vi "Get settings chain.vi"(8 "error in (no error)":errorcluster, 11 "ConfocalStageBase in":refnum<class "ConfocalStage.lvclass">) -> (0 "error out":errorcluster, 1 "class name":string[](array[string]), 2 "settings":variant[](array[variant]), 3 "ConfocalStageBase out":refnum<class "ConfocalStage.lvclass">)   [LabVIEW 2012, in "ConfocalStage.lvclass"]
doc: "Returns an array of variants containing the settings clusters of each class in the inheritance chain (lowest child class first), together with an array of all class names in the inheritance chain.\n\nFor classes without settings cluster, the settings chain contains empty variants."
uses:
  ConfocalStage.lvclass
  <vilib>/Distrio/Murmex/Murmex/Murmex.lvclass
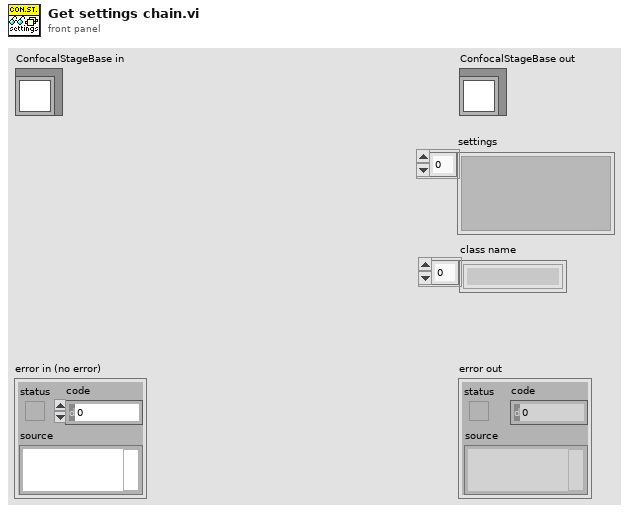
[diagram p1: front panel]
types:
  T1 = typedef "ConfocalStage.lvclass/settings.ctl" = cluster{"X stage speed":dbl, "Y stage speed":dbl, "Z stage speed":dbl}
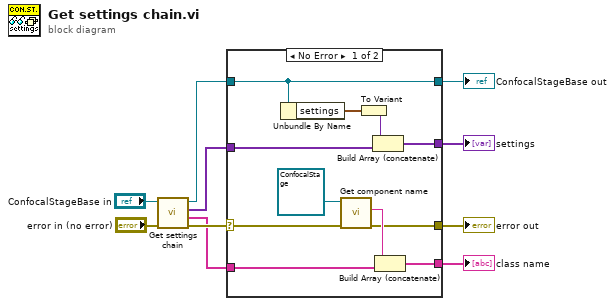
[diagram p0: block diagram]
diagram:
  n1 = call-parent "Get settings chain.vi"("error in (no error)"="error in (no error)", "MurmexBase in"="ConfocalStageBase in") -> ("error out"=w8:errorcluster, "class name"=w3:string[], "settings"=w4:variant[], "MurmexBase out"=w6:refnum<class "ConfocalStage.lvclass">)  [unwired: 6 in]
  n2 = case shown="No Error" w8 {
    selector: w8 -> [w18 w22]
    tunnel: [w17 w22] -> w7
    tunnel: w6 -> [w16 w23]
    tunnel: [w16 w23] -> w5
    tunnel: w4 -> [w15 _]
    tunnel: w3 -> [w14 _]
    tunnel: [w12 _] -> w2
    tunnel: [w11 _] -> w1
    frame No Error {
      n3 = Unbundle By Name(w16) -> ("settings"=w20:T1)
      n4 = call <vilib>:"Get component name.vi"("error in (no error)"=w18, "Murmex in"=refnum<class "ConfocalStage.lvclass"> refnum ("ConfocalStageBase in")) -> ("error out"=w17:errorcluster, "component name"=w19:string)  [unwired: 7 in, 1 out]
      n5 = To Variant(anything=w20) -> (Variant=w21:variant)
      n6 = Build Array (concatenate)(w21, w15) -> (w12:variant[])
      n7 = Build Array (concatenate)(w19, w14) -> (w11:string[])
    }
    frame Error {
    }
  }
  "error out" <- w7
  "ConfocalStageBase out" <- w5
  "settings" <- w2
  "class name" <- w1
